vi "GetSettings.vi"(8 "error in (no error)":errorcluster, 10 "SettingsToRetrieve":variant, 11 "ChromaAcLoad in":refnum<class "ChromaAcLoad.lvclass">) -> (0 "error out":errorcluster, 1 "DeviceConfig&Meas":variant, 2 "SettingsRetrieved":variant, 3 "ChromaAcLoad Out":refnum<class "ChromaAcLoad.lvclass">)   [LabVIEW 2018, in "AcPwrPlugins.lvlib" / "ChromaAcLoad.lvclass"]
doc: "This VI retrieves a boolean status to see if the instrument can conduct measurements while the device is changing modes or turning off and on."
uses:
  ChromaAcLoad.lvclass
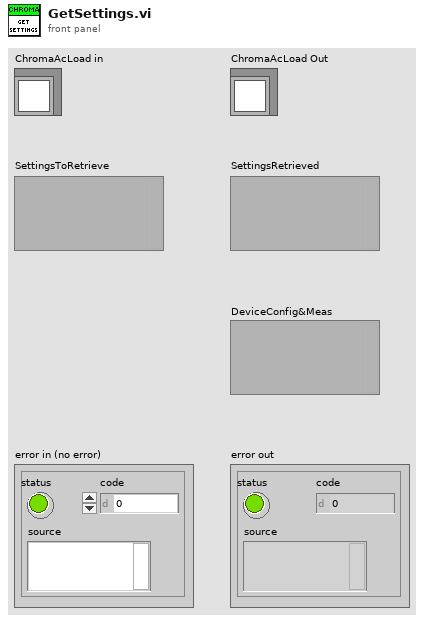
[diagram p1: front panel]
types:
  T1 = typedef "AcPwrPlugins.lvlib/ChromaAcLoad.lvclass/Device(s)Settings.ctl" = cluster{"Configuration Mode":enum16{"Constant Voltage (DC)", "Constant Power (DC)", "Constant Power (AC)", "Constant Current (DC)", "Constant Current (AC)", "Constant Resistance (DC)", "Constant Resistance (AC)", "Rectified Mode (DC)", "Inrush (AC)", "RLC CP (AC)", "RLC (AC)"}, "Phases":cluster{"Handle":string, "Name":string, "Phase Select":i32, "Instrument Options":string, "id query (T)":bool, "reset device (T)":bool, "Load Short Circuited":bool, "Line Synchronization":bool, "Load Current (A/Arms)":dbl, "Load Voltage (V/Vrms)":dbl, "Load Power (W)":dbl, "Load Resistance (Ohms)":dbl, "Load Current Peak Limit (A)":dbl, "Load Current Limit (A/Arms)":dbl, "Load Power Limit (W)":dbl, "Synch Frequency (Hz)":dbl, "Priority":enum16{"CF Only", "PF Only", "Both (CF)", "Both (PF)"}, "Crest Factor":dbl, "Power Factor":dbl, "Slew Rate":cluster{"Rise Slew Rate (A/ms)":i32, "Fall Slew Rate (A/ms)":i32}, "LC/RLC Mode":cluster{"Capacitance (uF)":i32, "Inductance (uH)":i32, "Series Resistance (Ohm)":dbl, "Parallel Resistance (Ohm)":dbl}, "Timing":cluster{"TimingOn":enum16{""}, "Hours":u32, "Minutes":u32, "Seconds":dbl, "CutoffVoltage":dbl}, "Connected":bool}[], "MeasName":string}
  T2 = typedef "AcPwrPlugins.lvlib/ChromaAcLoad.lvclass/Measurements.ctl" = cluster{"Handle":string, "Name":string, "Enabled":bool, "Measurement Value":dbl, "Hold Peak Current Measurement":bool, "btnMeasFetch":bool, "ProtectionStatusString":string, "Measurement Type":T3}[]
  T3 = typedef "AcPwrPlugins.lvlib/ChromaAcLoad.lvclass/MeasurementType.ctl" = enum16{"Voltage (Vrms or V)", "Current (Arms or A)", "Power (W)", "Peak Voltage (V)", "Peak Current (A)", "Peak Power (W)", "Frequency (Hz)", "Resistance (Ohms)", "Voltage Overshoot (V)", "Positive Peak Current (A)", "Voltage Undershoot (V)", "Negative Peak Current (A)", "Apparent Power (VA)", "Reacitive Power (VAR)", "Voltage THD", "Power Factor", "Current's Crest Factor"}
  T4 = cluster{"xml string":string, "xml string":string}
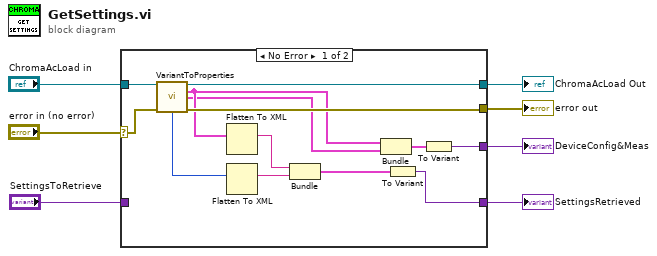
[diagram p0: block diagram]
diagram:
  n1 = case shown="No Error" "error in (no error)" {
    selector: "error in (no error)" -> [w20 w22]
    tunnel: "ChromaAcLoad in" -> [w19 w23]
    tunnel: [w18 w23] -> w5
    tunnel: [w12 w22] -> w4
    tunnel: "SettingsToRetrieve" -> [_ w21]
    tunnel: [w13 w21] -> w2
    tunnel: [w11 _] -> w1
    frame No Error {
      n2 = call "VariantToProperties.vi"("ChromaAcLoad"=w19, "error in (no error)"=w20) -> ("ChromaAcLoad"=w18:refnum<class "ChromaAcLoad.lvclass">, "Device Properties"=w10:T1, "Meas"=w9:T2, "Measurement Refresh Time (ms)"=w16:u32, "error out"=w12:errorcluster)  [unwired: 7 in, 2 out]
      n3 = Flatten To XML(anything=w10) -> (xml string=w15:string)
      n4 = Flatten To XML(anything=w16) -> (xml string=w14:string)
      n5 = Bundle("xml string"=w15, "xml string"=w14) -> (w17:T4)  [unwired: 1 in]
      n6 = Bundle("Device Properties"=w10, "Meas"=w9) -> (w8:cluster{"Device Properties":T1, "Meas":T2})  [unwired: 1 in]
      n7 = To Variant(anything=w17) -> (Variant=w13:variant)
      n8 = To Variant(anything=w8) -> (Variant=w11:variant)
    }
    frame Error {
    }
  }
  "error out" <- w4
  "ChromaAcLoad Out" <- w5
  "SettingsRetrieved" <- w2
  "DeviceConfig&Meas" <- w1
